vi "Set Attributes.vi"(8 "error in (no error)":errorcluster, 11 "Name Only Dialog in":refnum<class "Name Only Dialog.lvclass">) -> (0 "error out":errorcluster, 3 "Name Only Dialog out":refnum<class "Name Only Dialog.lvclass">)   [LabVIEW 2017, in "Name Only Dialog.lvclass"]
uses:
  Name Only Dialog.lvclass
  ITest Executive Builder Dialog/ITest Executive Builder Dialog.lvclass
  <vilib>/gpm_packages/@cs/test-executive/Source/Test Executive/TestExecutive Ref/TestExecutive Ref.lvclass
  C:/Users/jonmc/Documents/Git/Test Executive Builder/Source/Test Executive Builder Dialogs/ITest Executive Builder Dialog/ITest Executive Builder Dialog.lvclass
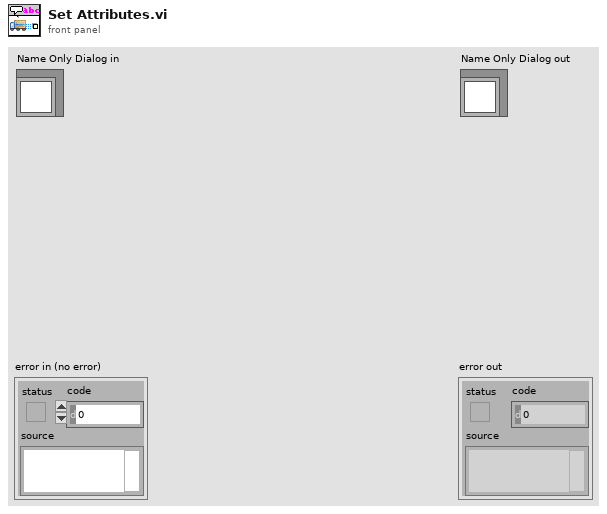
[diagram p1: front panel]
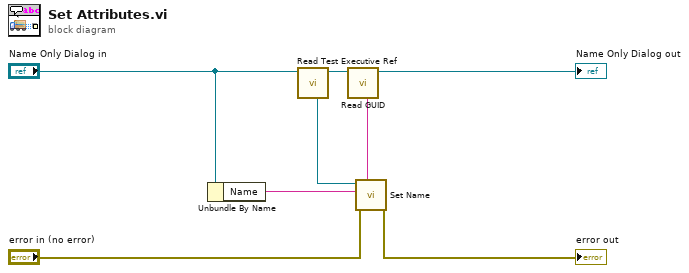
[diagram p0: block diagram]
diagram:
  n1 = Unbundle By Name("Name Only Dialog in") -> ("Name"=w5:string)
  n2 = call "Read Test Executive Ref.vi"("ITest Executive Builder Dialog in"="Name Only Dialog in") -> ("ITest Executive Builder Dialog out"=w8:refnum<class "Name Only Dialog.lvclass">, "Test Executive Ref"=w7:refnum<data-value>)  [unwired: 9 in]
  n3 = call "Read GUID.vi"("ITest Executive Builder Dialog in"=w8) -> ("ITest Executive Builder Dialog out"=→"Name Only Dialog out":refnum<class "Name Only Dialog.lvclass">, "GUID"=w6:string)  [unwired: 9 in]
  n4 = call <vilib>:"Set Name.vi"("Unique ID"=w6, "error in (no error)"="error in (no error)", "Name"=w5, "Test Executive Ref"=w7) -> ("error out"=→"error out":errorcluster)  [unwired: 6 in, 1 out]
